vi "RTS CVS Data Save.vi"(7 "Setup Info Station 9":string[][](array[string]), 8 "error in (no error)":errorcluster, 9 "Send Data":string[][](array[string]), 11 "TDMS File Location 8":path) -> (0 "error out":errorcluster, 3 "Path":path)   [LabVIEW 2016]
uses:
  <vilib>/Utility/file.llb/Write Delimited Spreadsheet (string).vi
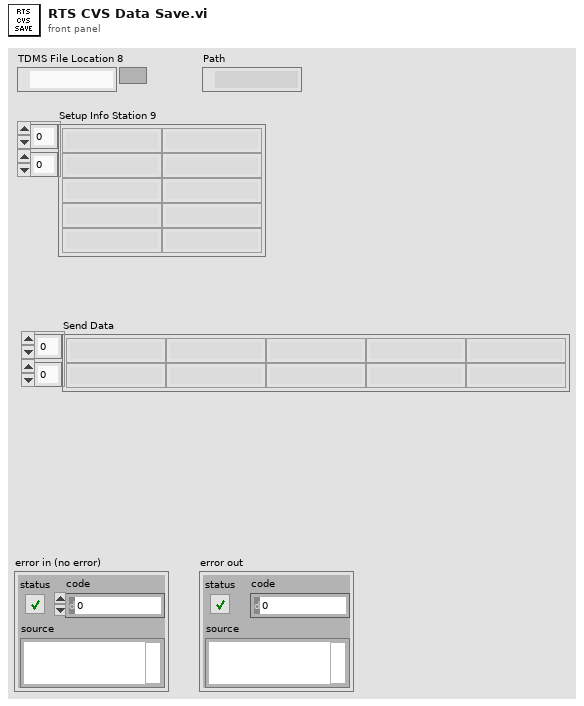
[diagram p1: front panel]
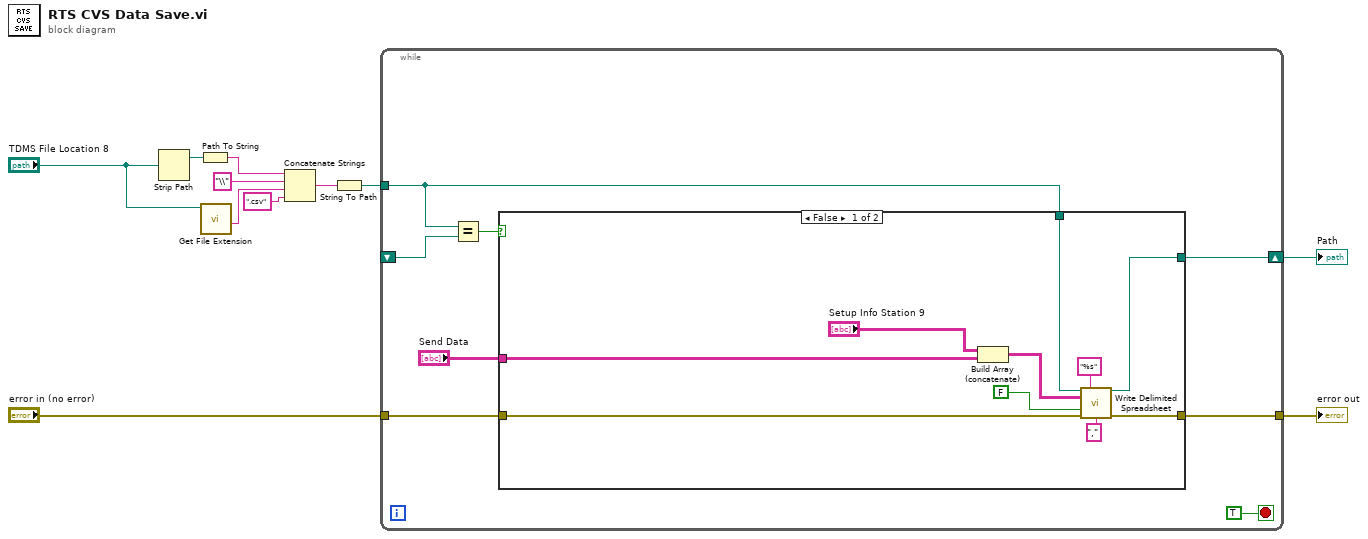
[diagram p0: block diagram]
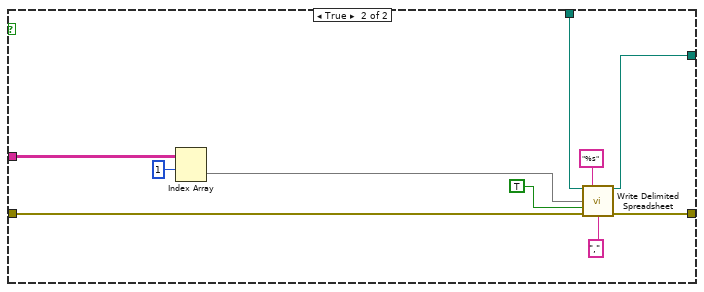
[diagram p2: hidden frame]
diagram:
  n1 = Strip Path(path="TDMS File Location 8") -> (stripped path=w7:path)  [unwired: 1 out]
  n2 = Path To String(path=w7) -> (string=w8:string)
  n3 = call <vilib>:"Get File Extension.vi"("file"="TDMS File Location 8") -> ("filename without extension"=w4:string)  [unwired: 6 in, 4 out]
  n4 = Concatenate Strings(w8, "\\" ("string"), w4, ".csv" ("string")) -> (w6:string)
  n5 = String To Path(string=w6) -> (path=w3:path)
  n6 = while {
    tunnel: [w19] -> w10
    shift-right: [w18] -> w11
    shift-left: _ -> [w16]
    tunnel: w3 -> [w17]
    tunnel: "error in (no error)" -> [w13]
    stop <- TRUE stop-if-true
    n7 = Equal?(x=w17, y=w16) -> (x = y?=w15:bool)
    n8 = case shown="False" w15 {
      tunnel: [w21 w39] -> w19
      tunnel: [w28 w34] -> w18
      tunnel: w17 -> [w29 w33]
      tunnel: "Send Data" -> [w23 w32]
      tunnel: w13 -> [w25 w31]
      frame False {
        n9 = Build Array (concatenate)("Setup Info Station 9", w23) -> (w22:string[][])
        n10 = call-poly <vilib>:"Write Delimited Spreadsheet.vi"("file path (dialog if empty)"=w29, "format (%s)"="%s" ("format (%.3f)"), "2D data"=w22, "append to file? (new file:F)"=FALSE, "error in (no error)"=w25, "delimiter (\\t)"="," ("delimiter (\\t)")) -> ("new file path (Not A Path if cancelled)"=w28:path, "error out"=w21:errorcluster)  [unwired: 8 in]
      }
      frame True {
        n11 = Index Array(array=w32, index (row)=1) -> (element=w37:string[])  [unwired: 1 in]
        n12 = call-poly <vilib>:"Write Delimited Spreadsheet.vi"("file path (dialog if empty)"=w33, "format (%s)"="%s", "1D data"=w37, "append to file? (new file:F)"=TRUE, "error in (no error)"=w31, "delimiter (\\t)"="," ("delimiter (\\t)")) -> ("new file path (Not A Path if cancelled)"=w34:path, "error out"=w39:errorcluster)  [unwired: 8 in]
      }
    }
  }
  "Path" <- w11
  "error out" <- w10
